vi "Get Path Commands.vi"(1 "Commands Raw Data":string) -> (0 "Commands":T1(array[cluster]))   [LabVIEW 2019]
doc: "This VI takes in raw path data and outputs an array of all the commands found."
uses:
  <vilib>/Utility/error.llb/whitespace.ctl
  <vilib>/regexp/Match Regular Expression.xnode
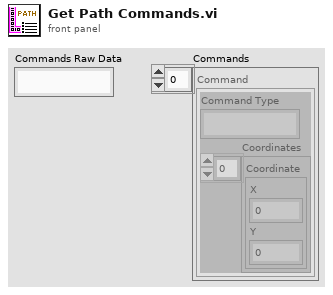
[diagram p1: front panel]
types:
  T1 = cluster{"Command Type":string, "Coordinates":cluster{"X":dbl, "Y":dbl}[]}[]
  T2 = typedef "whitespace.ctl" = u16
  T3 = cluster{"submatch 1":string, cluster{dbl, dbl}[]}
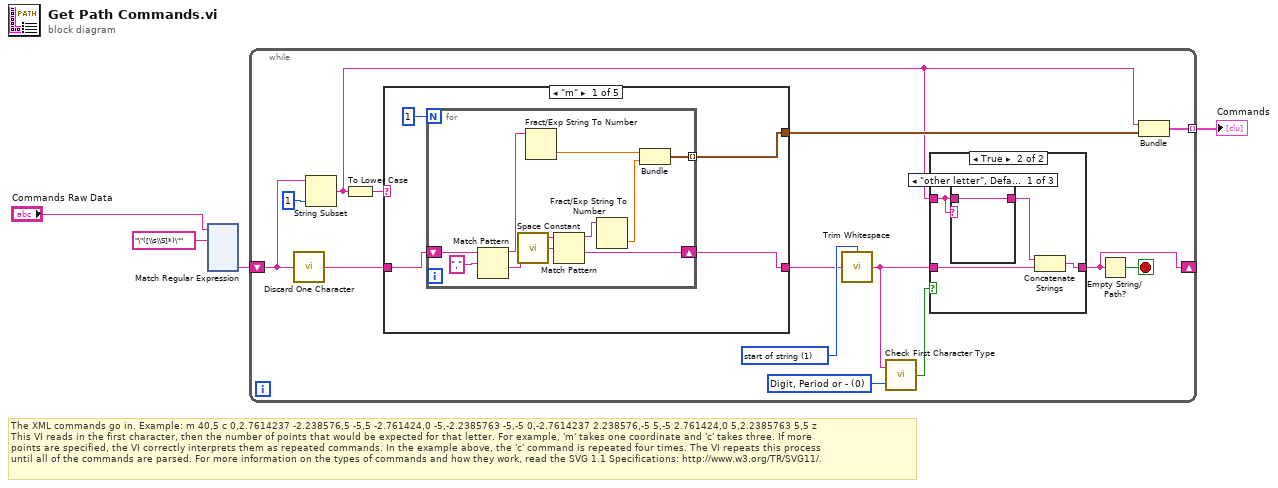
[diagram p0: block diagram]
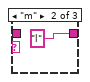
[diagram p3: hidden frame]
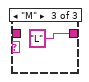
[diagram p4: hidden frame]
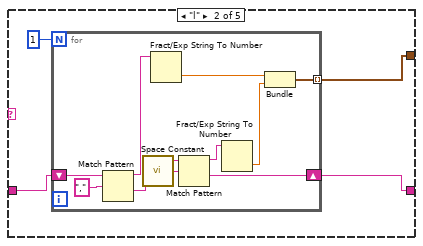
[diagram p5: hidden frame]
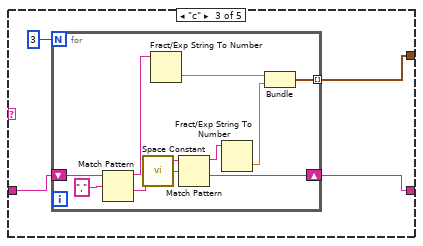
[diagram p6: hidden frame]
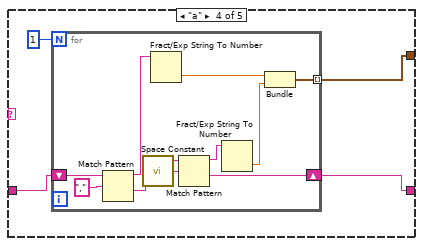
[diagram p7: hidden frame]
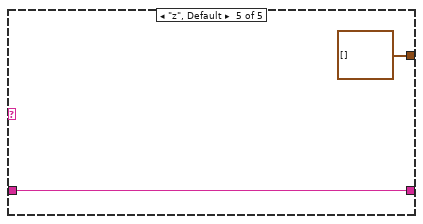
[diagram p8: hidden frame]
diagram:
  # "The XML commands go in. Example: m 40,5 c 0,2.7614237 -2.238576,5 -5,5 -2.761424,0 -5,-2.2385763 -5,-5 0,-2.7614237 2.238576,-5 5,-5 2.761424,0 5,2.2385763 5,5 z\nThis VI reads in the first character, then the number of points that would be expected for that letter. For example, 'm' takes one coordinate and 'c' takes three. If more\npoints are specified, the VI correctly interprets them as repeated commands. In the example above, the 'c' command is repeated four times. The VI repeats this process\nuntil all of the commands are parsed. For more information on the types of commands and how they work, read the SVG 1.1 Specifications: http://www.w3.org/TR/SVG11/."
  n1 = xnode "Match Regular Expression"("input string"="Commands Raw Data", "regular expression"="\"([\\s\\S]*)\"") -> ("submatch 1"=w2:string)  [unwired: 4 in, 5 out]
  n2 = while {
    shift-right: [w5] -> _
    shift-left: w2 -> [w7]
    tunnel: [w14] -> w4 mode=indexing
    stop <- w17 stop-if-true
    w11 = u16 0 items=["Digit, Period or -", "\"", "Character", "Space or Comma"] ("Type")
    w13 = T2 1 items=["both", "start of string", "end of string"] ("location (both)")
    n3 = call "Discard One Character.vi"("String"=w7) -> ("Remaining String"=w6:string)
    n4 = String Subset(string=w7, length (rest)=1 ("length (rest)")) -> (substring=w8:string)  [unwired: 1 in]
    n5 = To Lower Case(string=w8) -> (all lower case string=w15:string)
    n6 = case shown="\"m\"" w15 {
      tunnel: [w29 w43 w57 w71 cluster{dbl, dbl}[] []] -> w16
      tunnel: w6 -> [w28 w42 w56 w70 w83]
      tunnel: [w27 w41 w55 w69 w83] -> w12
      frame "m" {
        n7 = for {
          N: 1 -> [_]
          tunnel: [w32] -> w29 mode=indexing
          shift-right: [w31] -> w27
          shift-left: w28 -> [w39]
          n8 = Match Pattern(string=w39, regular expression=",") -> (before substring=w38:string, after substring=w37:string)  [unwired: 1 in, 2 out]
          n9 = call <vilib>:"Space Constant.vi"() -> ("String"=w36:string)
          n10 = Fract/Exp String To Number(string=w38) -> (number=w33:dbl)  [unwired: 3 in, 1 out]
          n11 = Match Pattern(string=w37, regular expression=w36) -> (before substring=w35:string, after substring=w31:string)  [unwired: 1 in, 2 out]
          n12 = Fract/Exp String To Number(string=w35) -> (number=w34:dbl)  [unwired: 3 in, 1 out]
          n13 = Bundle(w33, w34) -> (w32:cluster{dbl, dbl})  [unwired: 1 in]
        }
      }
      frame "l" {
        n14 = for {
          N: 1 -> [_]
          tunnel: [w46] -> w43 mode=indexing
          shift-right: [w45] -> w41
          shift-left: w42 -> [w53]
          n15 = Match Pattern(string=w53, regular expression=",") -> (before substring=w52:string, after substring=w51:string)  [unwired: 1 in, 2 out]
          n16 = call <vilib>:"Space Constant.vi"() -> ("String"=w50:string)
          n17 = Fract/Exp String To Number(string=w52) -> (number=w47:dbl)  [unwired: 3 in, 1 out]
          n18 = Match Pattern(string=w51, regular expression=w50) -> (before substring=w49:string, after substring=w45:string)  [unwired: 1 in, 2 out]
          n19 = Fract/Exp String To Number(string=w49) -> (number=w48:dbl)  [unwired: 3 in, 1 out]
          n20 = Bundle(w47, w48) -> (w46:cluster{dbl, dbl})  [unwired: 1 in]
        }
      }
      frame "c" {
        n21 = for {
          N: 3 -> [_]
          tunnel: [w60] -> w57 mode=indexing
          shift-right: [w59] -> w55
          shift-left: w56 -> [w67]
          n22 = Match Pattern(string=w67, regular expression=",") -> (before substring=w66:string, after substring=w65:string)  [unwired: 1 in, 2 out]
          n23 = call <vilib>:"Space Constant.vi"() -> ("String"=w64:string)
          n24 = Fract/Exp String To Number(string=w66) -> (number=w61:dbl)  [unwired: 3 in, 1 out]
          n25 = Match Pattern(string=w65, regular expression=w64) -> (before substring=w63:string, after substring=w59:string)  [unwired: 1 in, 2 out]
          n26 = Fract/Exp String To Number(string=w63) -> (number=w62:dbl)  [unwired: 3 in, 1 out]
          n27 = Bundle(w61, w62) -> (w60:cluster{dbl, dbl})  [unwired: 1 in]
        }
      }
      frame "a" {
        n28 = for {
          N: 1 -> [_]
          tunnel: [w74] -> w71 mode=indexing
          shift-right: [w73] -> w69
          shift-left: w70 -> [w81]
          n29 = Match Pattern(string=w81, regular expression=",") -> (before substring=w80:string, after substring=w79:string)  [unwired: 1 in, 2 out]
          n30 = call <vilib>:"Space Constant.vi"() -> ("String"=w78:string)
          n31 = Fract/Exp String To Number(string=w80) -> (number=w75:dbl)  [unwired: 3 in, 1 out]
          n32 = Match Pattern(string=w79, regular expression=w78) -> (before substring=w77:string, after substring=w73:string)  [unwired: 1 in, 2 out]
          n33 = Fract/Exp String To Number(string=w77) -> (number=w76:dbl)  [unwired: 3 in, 1 out]
          n34 = Bundle(w75, w76) -> (w74:cluster{dbl, dbl})  [unwired: 1 in]
        }
      }
      frame "z", Default {
      }
    }
    n35 = call <vilib>:"Trim Whitespace.vi"("string"=w12, "location (both)"=w13) -> ("trimmed string"=w9:string)
    n36 = call "Check First Character Type.vi"("Type"=w11, "Character"=w9) -> ("True/False"=w10:bool)
    n37 = case shown="True" w10 {
      tunnel: w9 -> [w19 w21]
      tunnel: w8 -> [_ w23]
      tunnel: [w19 w20] -> w5
      frame False {
      }
      frame True {
        n38 = case shown="\"other letter\", Default" w23 {
          tunnel: w23 -> [w24 _ _]
          tunnel: [w24 "l" "L"] -> w22
          frame "other letter", Default {
          }
          frame "m" {
          }
          frame "M" {
          }
        }
        n39 = Concatenate Strings(w22, w21) -> (w20:string)
      }
    }
    n40 = Empty String/Path?(string/path=w5) -> (empty?=w17:bool)
    n41 = Bundle("submatch 1"=w8, w16) -> (w14:T3)  [unwired: 1 in]
  }
  "Commands" <- w4
